vi "moving average (subVI).vi"(10 "average num":u16, 11 "Array in":dbl[](array[numeric])) -> (3 "Array out":dbl[](array[numeric]))   [LabVIEW 2024]
uses:
  <vilib>/Analysis/baseanly.llb/Mean (DBL).vi
  <vilib>/Analysis/NI_AALBase.lvlib
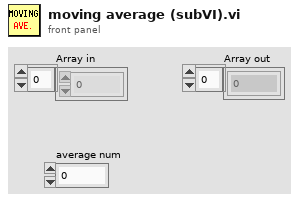
[diagram p1: front panel]
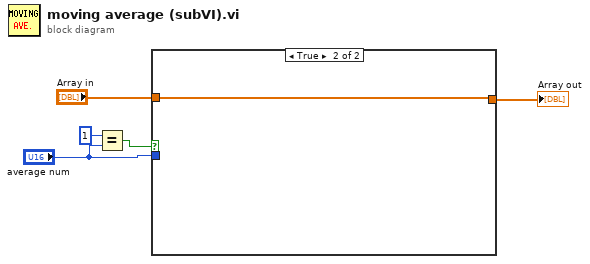
[diagram p0: block diagram]
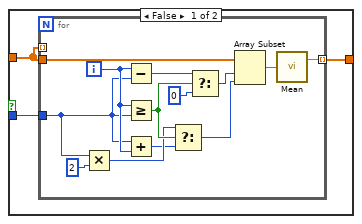
[diagram p2: hidden frame]
diagram:
  n1 = Equal?(x=u16 1, y="average num") -> (x = y?=w1:bool)
  n2 = case shown="True" w1 {
    tunnel: [w8 w22] -> w5
    tunnel: "Array in" -> [w7 w22]
    tunnel: "average num" -> [w6 _]
    frame False {
      n3 = for {
        tunnel: w7 -> [_] mode=indexing
        tunnel: w7 -> [w21]
        tunnel: w6 -> [w9]
        tunnel: [w19] -> w8 mode=indexing
        i -> [w11]
        n4 = Multiply(x=w9, y=u16 2) -> (x*y=w12:u16)
        n5 = Subtract(x=w11, y=w9) -> (x-y=w15:i32)
        n6 = Greater Or Equal?(x=w11, y=w9) -> (x >= y?=w16:bool)
        n7 = Add(x=w9, y=w11) -> (x+y=w10:i32)
        n8 = Select(t=w12, s=w16, f=w10) -> (s? t:f=w18:i32)
        n9 = Select(t=w15, s=w16, f=0) -> (s? t:f=w14:i32)
        n10 = Array Subset(array=w21, index=w14, length=w18) -> (w20:dbl[])
        n11 = call-poly <vilib>:"Mean.vi"("X"=w20) -> ("mean"=w19:dbl)  [unwired: 1 out]
      }
    }
    frame True {
    }
  }
  "Array out" <- w5
